vi "torque - read all files V1.vi"(6 "Numeric Control":i32, 7 "container action":T3, 8 "hash key":T2, 9 "torque -- hash value IN":T1={"time (sec) array"=[], "temperature (K) array"=[], "SRS Vx (V) array"=[], "field (T) array"=[], "filename"="name", "time OK?"=FALSE, "temperature OK?"=FALSE, "SRS OK?"=FALSE, "FIELD OK?"=FALSE}, 10 "filename":string="30K_-45D_001_061513.dat", 11 "folder Path":path=path "C:/Users/224586/Downloads/arkady/Torque-Jun2013/rotationset5/30K") -> (1 "torque -- hash value OUT":T1={"time (sec) array"=[], "temperature (K) array"=[], "SRS Vx (V) array"=[], "field (T) array"=[], "filename"="name", "time OK?"=FALSE, "temperature OK?"=FALSE, "SRS OK?"=FALSE, "FIELD OK?"=FALSE}, 3 "OK?":bool)   [LabVIEW 2012]
uses:
  container action.ctl
  torque -- hash key.ctl
  torque -- hash value.ctl
  hash action control.ctl
  torque -- filename action.ctl
  hash action stack.vi
  file - read list of lines.vi
  parse - find tokens.vi
  array -- fold to mon increasing.vi
  parse -- get list of matches -- numbers.vi
panel:
  out "Key table OUT":T2[](array[typedef])
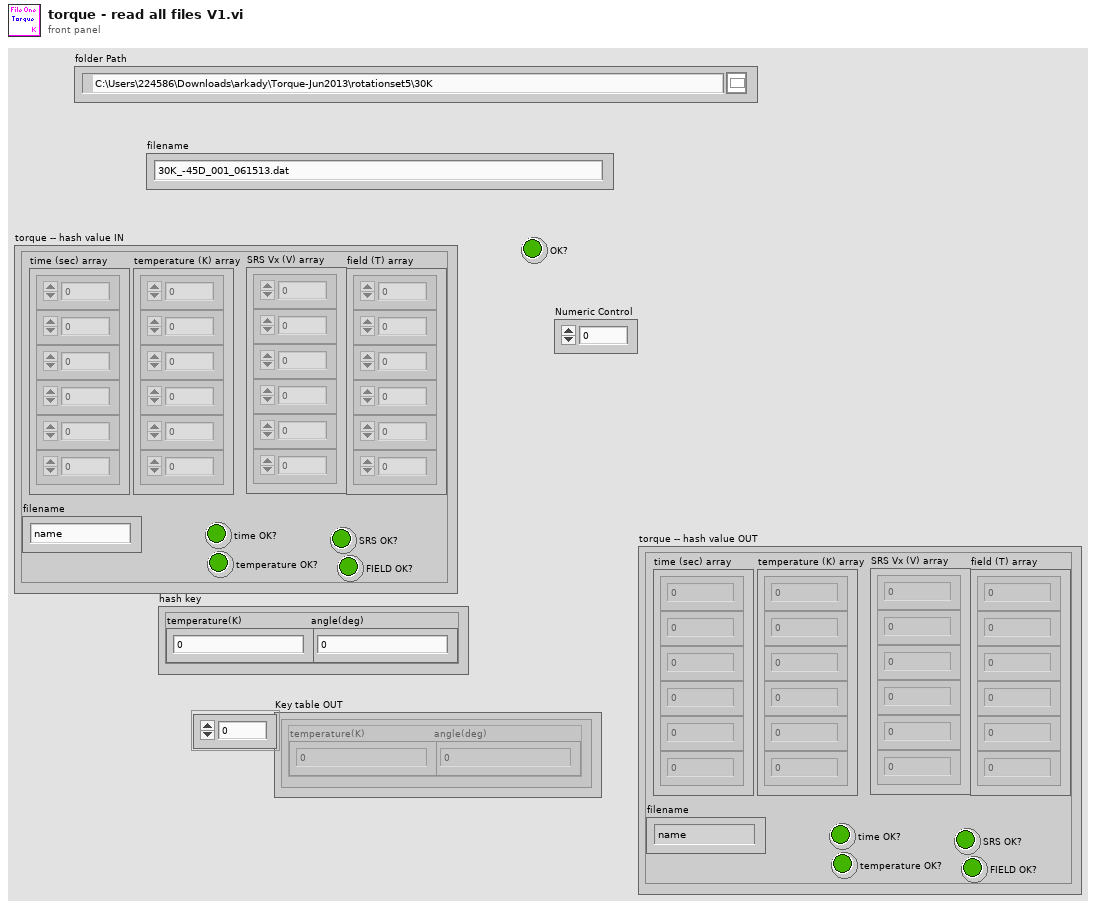
[diagram p1: front panel]
types:
  T1 = typedef "torque -- hash value.ctl" = cluster{"time (sec) array":dbl[], "temperature (K) array":dbl[], "SRS Vx (V) array":dbl[], "field (T) array":dbl[], "filename":string, "time OK?":bool, "temperature OK?":bool, "SRS OK?":bool, "FIELD OK?":bool}
  T2 = typedef "torque -- hash key.ctl" = cluster{"temperature(K)":dbl, "angle(deg)":dbl}
  T3 = typedef "container action.ctl" = enum16{"get", "read file", "plot", "init", "set"}
  T4 = typedef "hash action control.ctl" = enum16{"get", "new", "--void", "delete", "delete all", "set", "--delete if exists", "--create if not there", "list keys", "index forw", "index back", "check", "index set", "find key"}
  T5 = typedef "torque -- filename action.ctl" = enum16{"parse", "build", "check"}
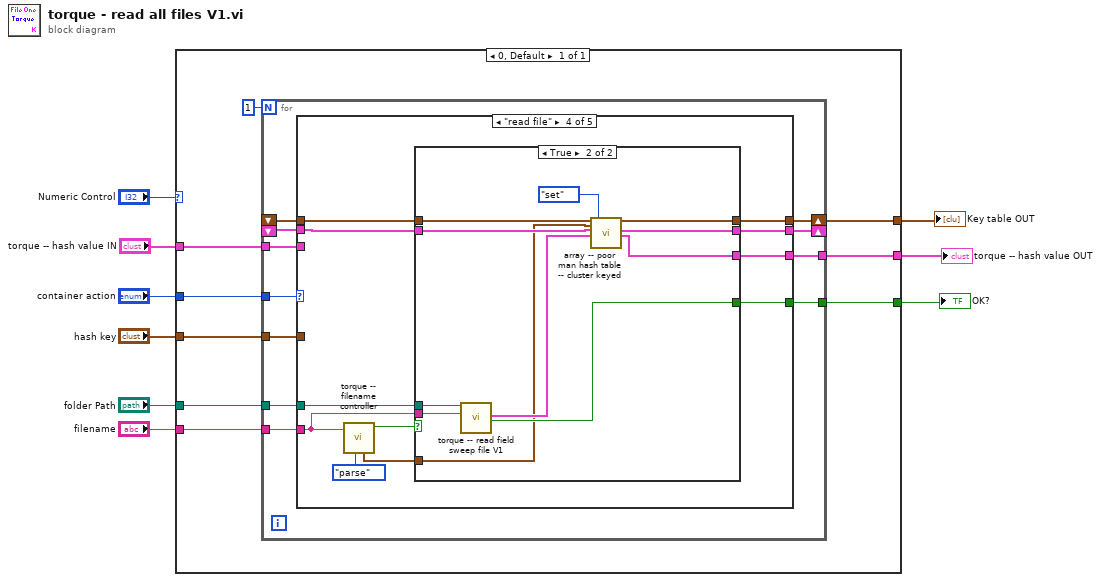
[diagram p0: block diagram]
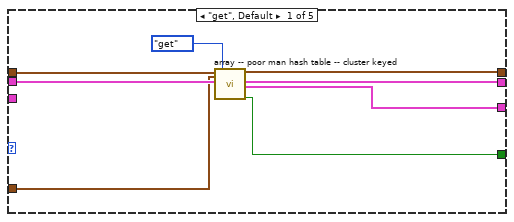
[diagram p2: hidden frame]
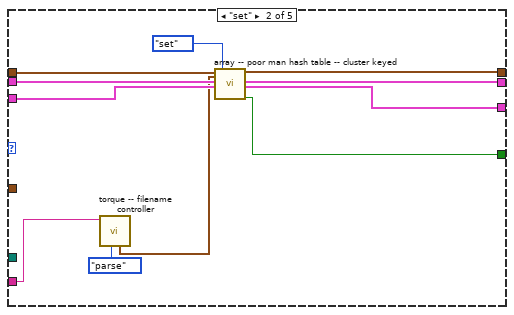
[diagram p3: hidden frame]
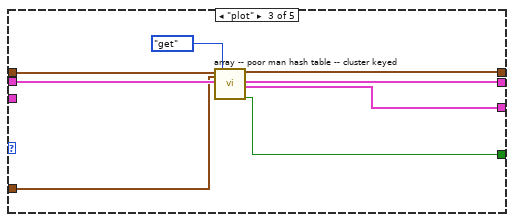
[diagram p4: hidden frame]
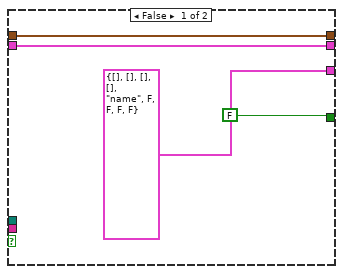
[diagram p5: hidden frame]
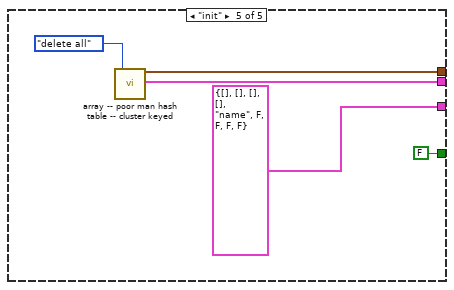
[diagram p6: hidden frame]
diagram:
  n1 = case shown="0, Default" "Numeric Control" {
    tunnel: [w15] -> w7
    tunnel: "folder Path" -> [w17]
    tunnel: "container action" -> [w16]
    tunnel: "filename" -> [w14]
    tunnel: "hash key" -> [w13]
    tunnel: [w12] -> w2
    tunnel: [w11] -> w3
    tunnel: "torque -- hash value IN" -> [w10]
    frame 0, Default {
      n2 = for {
        N: 1 -> [_]
        tunnel: w17 -> [w29]
        tunnel: w16 -> [w28]
        tunnel: [w27] -> w15
        tunnel: w14 -> [w26]
        shift-right: [w25] -> w12
        shift-left: _ -> [w23]
        shift-right: [w24] -> _
        shift-left: _ -> [w22]
        tunnel: w13 -> [w21]
        tunnel: [w20] -> w11
        tunnel: w10 -> [w19]
        n3 = case shown="\"read file\"" w28 {
          tunnel: [w32 w43 w51 w66 FALSE ("OK?")] -> w27
          tunnel: w29 -> [_ _ _ w67 _]
          tunnel: w26 -> [_ w39 _ w59 _]
          tunnel: [w36 w47 w55 w63 w87] -> w25
          tunnel: [w34 w45 w53 w60 w86] -> w24
          tunnel: w23 -> [w37 w48 w56 w62 _]
          tunnel: w22 -> [w35 w46 w54 w61 _]
          tunnel: w21 -> [w31 _ w50 _ _]
          tunnel: [w30 w42 w49 w58 T1 {"time (sec) array"=[], "temperature (K) array"=[], "SRS Vx (V) array"=[], "field (T) array"=[], "filename"="name", "time OK?"=FALSE, "temperature OK?"=FALSE, "SRS OK?"=FALSE, "FIELD OK?"=FALSE} ("torque -- hash value OUT")] -> w20
          tunnel: w19 -> [_ w41 _ _ _]
          frame "get", Default {
            n4 = call "array -- poor man hash table -- cluster keyed .vi"("key table"=w37, "hash key"=w31, "value table"=w35, "hash action"=hash_action_control."get") -> ("Key table OUT"=w36:T2[], "value table OUT"=w34:T1[], "torque -- hash value OUT"=w30:T1, "found?"=w32:bool)  [unwired: 10 in, 2 out]
          }
          frame "set" {
            n5 = call "torque -- filename controller.vi"("filename action"=torque_--_filename_action."parse", "String"=w39) -> ("hash key"=w38:T2)  [unwired: 5 in, 4 out]
            n6 = call "array -- poor man hash table -- cluster keyed .vi"("key table"=w48, "hash key"=w38, "value table"=w46, "torque -- hash value"=w41, "hash action"=hash_action_control."set") -> ("Key table OUT"=w47:T2[], "value table OUT"=w45:T1[], "torque -- hash value OUT"=w42:T1, "found?"=w43:bool)  [unwired: 9 in, 2 out]
          }
          frame "plot" {
            n7 = call "array -- poor man hash table -- cluster keyed .vi"("key table"=w56, "hash key"=w50, "value table"=w54, "hash action"=hash_action_control."get") -> ("Key table OUT"=w55:T2[], "value table OUT"=w53:T1[], "torque -- hash value OUT"=w49:T1, "found?"=w51:bool)  [unwired: 10 in, 2 out]
          }
          frame "read file" {
            n8 = call "torque -- filename controller.vi"("filename action"=torque_--_filename_action."parse", "String"=w59) -> ("Ok?"=w64:bool, "hash key"=w57:T2)  [unwired: 5 in, 3 out]
            n9 = case shown="True" w64 {
              tunnel: w67 -> [_ w77]
              tunnel: [FALSE w82] -> w66
              tunnel: [w71 w81] -> w63
              tunnel: w62 -> [w71 w80]
              tunnel: w61 -> [w69 w79]
              tunnel: [w69 w78] -> w60
              tunnel: w59 -> [_ w76]
              tunnel: [T1 {"time (sec) array"=[], "temperature (K) array"=[], "SRS Vx (V) array"=[], "field (T) array"=[], "filename"="name", "time OK?"=FALSE, "temperature OK?"=FALSE, "SRS OK?"=FALSE, "FIELD OK?"=FALSE} ("torque -- hash value OUT") w73] -> w58
              tunnel: w57 -> [_ w72]
              frame False {
              }
              frame True {
                n10 = call "torque -- read field sweep file V1.vi"("folder path"=w77, "filename"=w76) -> ("torque -- hash value"=w74:T1, "OK?"=w82:bool)  [unwired: 16 in]
                n11 = call "array -- poor man hash table -- cluster keyed .vi"("key table"=w80, "hash key"=w72, "value table"=w79, "torque -- hash value"=w74, "hash action"=hash_action_control."set") -> ("Key table OUT"=w81:T2[], "value table OUT"=w78:T1[], "torque -- hash value OUT"=w73:T1)  [unwired: 9 in, 3 out]
              }
            }
          }
          frame "init" {
            n12 = call "array -- poor man hash table -- cluster keyed .vi"("hash action"=hash_action_control."delete all") -> ("Key table OUT"=w87:T2[], "value table OUT"=w86:T1[])  [unwired: 13 in, 4 out]
          }
        }
      }
    }
  }
  "OK?" <- w7
  "torque -- hash value OUT" <- w3
  "Key table OUT" <- w2
